vi "Save File HEWH Create Save Directory.vi"(8 "error in (no error)":errorcluster, 9 "Lab ID":string, 10 "TR Number":string, 11 "FileName DataLog":path) -> (0 "error out":errorcluster, 3 "File Path":path)   [LabVIEW 2016, in "File Setup.lvlib"]
uses:
  File Setup.lvlib
panel:
  out "match substring":string
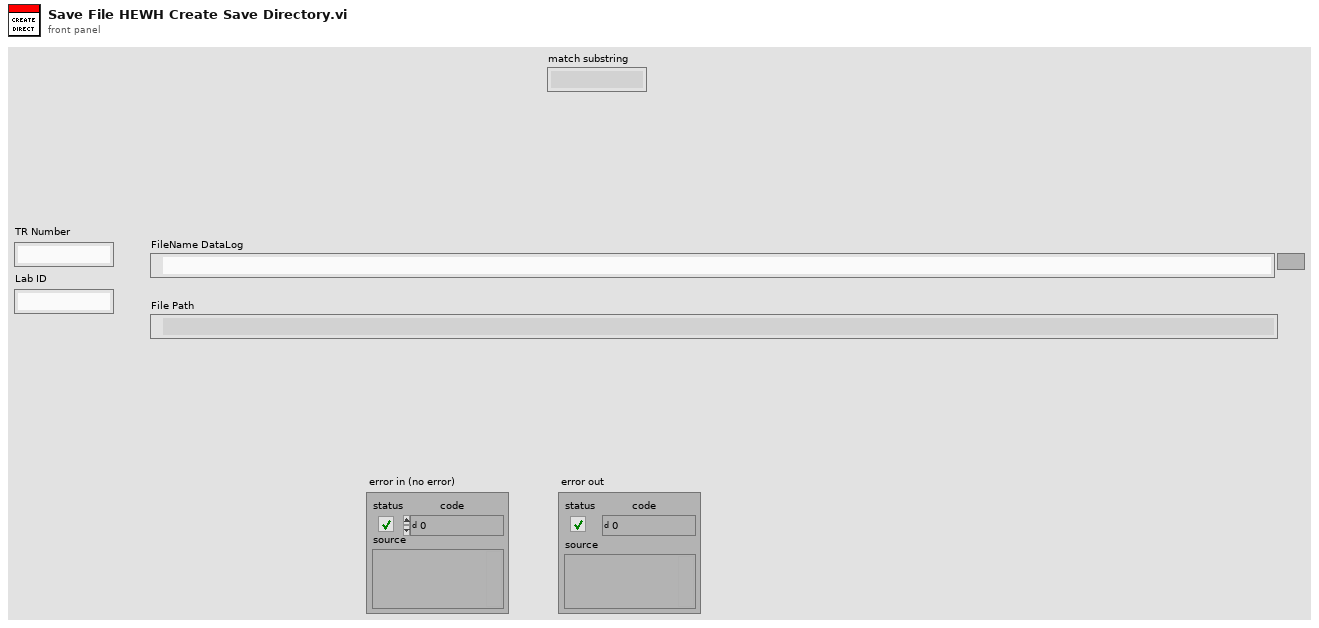
[diagram p1: front panel]
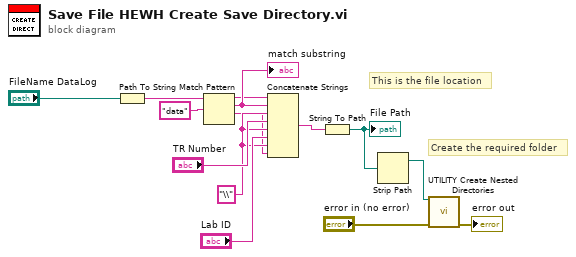
[diagram p0: block diagram]
diagram:
  w4 = "\\"
  # "This is the file location"
  # "Create the required folder"
  n1 = Path To String(path="FileName DataLog") -> (string=w13:string)
  n2 = Match Pattern(string=w13, regular expression="data") -> (before substring=w8:string, match substring=w11:string, after substring=w3:string)  [unwired: 1 in, 1 out]
  "match substring" <- w11
  n3 = Concatenate Strings(w8, w11, w4, "TR Number", w4, "Lab ID", w4, w3) -> (w7:string)
  n4 = String To Path(string=w7) -> (path=w6:path)
  "File Path" <- w6
  n5 = Strip Path(path=w6) -> (stripped path=w5:path)  [unwired: 1 out]
  n6 = call "UTILITY Create Nested Directories.vi"("path to create"=w5, "error in"="error in (no error)") -> ("error out"=→"error out":errorcluster)  [unwired: 11 in, 2 out]
